vi "AQT_initialize.vi"() -> (2 "function returns":u32[](array[numeric]), 3 "hnd out":u32)   [LabVIEW 2013]
panel:
  in  "Path":path=path "C:/Users/QC/Documents/Cesium_project/LabVIEW Projects/Cesium_control/cesium_controller_stable/cesium_controller/AQT_MEMS_switch/interface.bit"
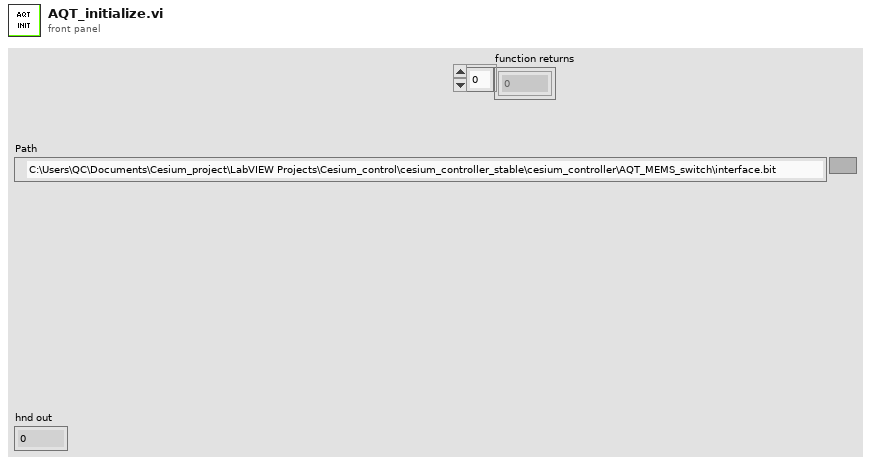
[diagram p1: front panel]
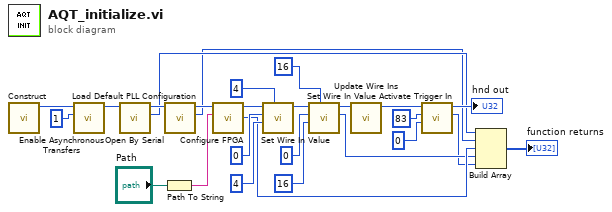
[diagram p0: block diagram]
diagram:
  n1 = call <userlib>:"Construct.vi"() -> ("function return"=w26:u32)  [unwired: 11 in]
  n2 = call <userlib>:"Enable Asynchronous Transfers.vi"("enable"=1, "hnd"=w26) -> ("hnd out"=w25:u32)  [unwired: 9 in]
  n3 = call <userlib>:"Open By Serial.vi"("hnd"=w25) -> ("function return"=w6:u32, "hnd out"=w24:u32)  [unwired: 9 in]
  n4 = Path To String(path="Path") -> (string=w8:string)
  n5 = call <userlib>:"Load Default PLL Configuration.vi"("hnd"=w24) -> ("function return"=w5:u32, "hnd out"=w23:u32)  [unwired: 9 in]
  n6 = call <userlib>:"Configure FPGA.vi"("strFilename"=w8, "hnd"=w23) -> ("function return"=w4:u32, "hnd out"=w10:u32)  [unwired: 8 in]
  n7 = call <userlib>:"Set Wire In Value.vi"("mask"=u32 4, "val"=u32 4, "ep"=0, "hnd"=w10) -> ("hnd out"=w14:u32)  [unwired: 6 in, 1 out]
  n8 = call <userlib>:"Set Wire In Value.vi"("mask"=u32 16, "val"=u32 16, "ep"=0, "hnd"=w14) -> ("function return"=w3:u32, "hnd out"=w15:u32)  [unwired: 6 in]
  n9 = call <userlib>:"Update Wire Ins.vi"("hnd"=w15) -> ("hnd out"=w21:u32)  [unwired: 10 in]
  n10 = call <userlib>:"Activate Trigger In.vi"("bit"=0, "epAddr"=83, "hnd"=w21) -> ("function return"=w2:u32, "hnd out"=→"hnd out":u32)  [unwired: 7 in]
  n11 = Build Array(w6, w5, w4, w3, w2) -> (→"function returns":u32[])
